vi "ZhuanVbeishu.vi"(11 "电压倍数":string) -> (2 "电压范围":string, 3 "最大电压值":i32)   [LabVIEW 2014, in "Sample.lvlib"]
uses:
  Sample/Sample.lvlib
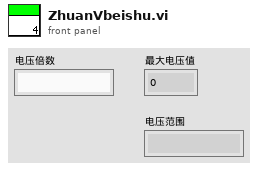
[diagram p1: front panel]
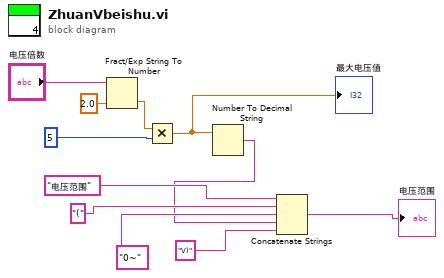
[diagram p0: block diagram]
diagram:
  n1 = Fract/Exp String To Number(string="电压倍数", default (0 dbl)=2.0 ("默认(0 DBL)")) -> (number=w4:dbl)  [unwired: 2 in, 1 out]
  n2 = Multiply(x=w4, y=5) -> (x*y=w2:dbl)
  "最大电压值" <- w2
  n3 = Number To Decimal String(number=w2) -> (decimal integer string=w1:string)  [unwired: 1 in]
  n4 = Concatenate Strings("电压范围", "(", "0~", w1, "V)") -> (→"电压范围":string)
